vi "Setup.vi"(8 "error in (no error)":errorcluster, 11 "Process Test In":refnum<class "Worker Test.lvclass">) -> (0 "error out":errorcluster, 3 "Process Test Out":refnum<class "Worker Test.lvclass">)   [LabVIEW 2020, in "Worker Test.lvclass"]
uses:
  Worker Test.lvclass
  C:/git/astemes-triarc-examples/source/Coffee Shop/Tests/Person Test/Person Test.lvclass
  Processes/People/Workers/Worker/Worker.lvclass
  C:/git/astemes-triarc-examples/source/Coffee Shop/Processes/People/Person/Person.lvclass
  Person Test/Person Test.lvclass
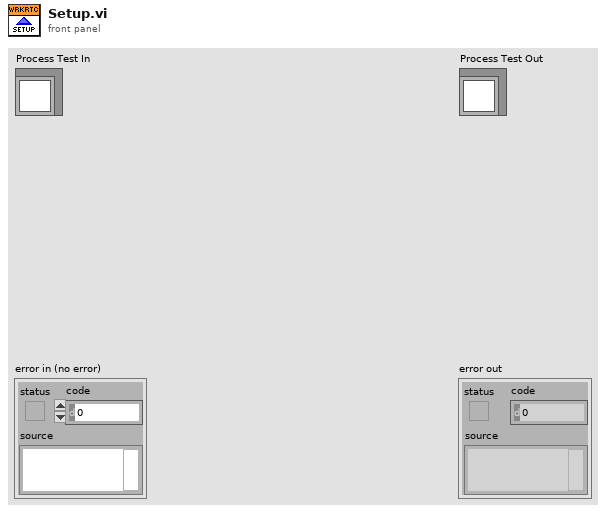
[diagram p1: front panel]
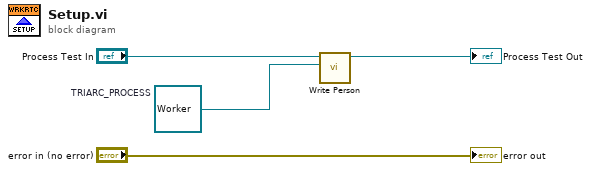
[diagram p0: block diagram]
diagram:
  w2 = refnum<class "Worker.lvclass"> refnum  # TRIARC_PROCESS
  n1 = call "Write Person.vi"("TRIARC_PROCESS"=w2, "Person Test in"="Process Test In") -> ("Person Test out"=→"Process Test Out":refnum<class "Worker Test.lvclass">)  [unwired: 9 in]
  "error out" <- "error in (no error)"
